vi "Write SA Pin.vi"(8 "error in (no error)":errorcluster, 10 "SA Pin":string, 11 "TDSCDMA_SEM in":refnum<class "TDSCDMA_SEM.lvclass">=refnum) -> (0 "error out":errorcluster, 3 "TDSCDMA_SEM out":refnum<class "TDSCDMA_SEM.lvclass">)   [LabVIEW 2016, in "SeqAuto Evaluations.lvlib" / "TDSCDMA_SEM.lvclass"]
uses:
  TDSCDMA_SEM.lvclass
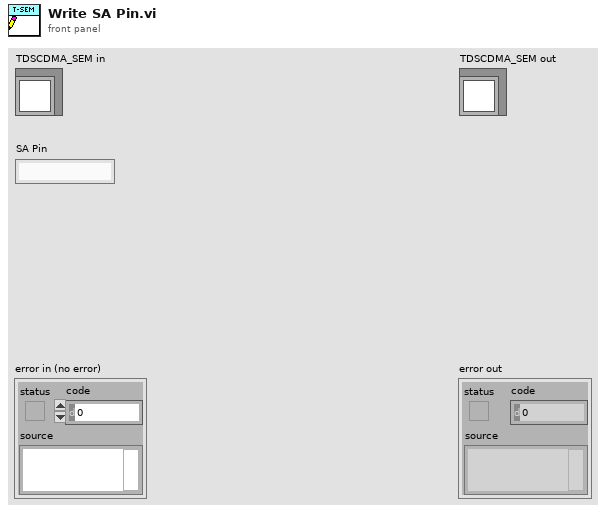
[diagram p1: front panel]
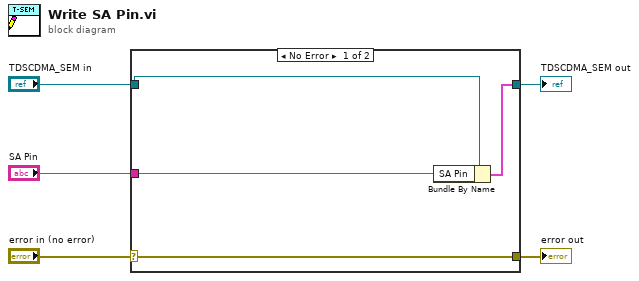
[diagram p0: block diagram]
diagram:
  n1 = case shown="No Error" "error in (no error)" {
    selector: "error in (no error)" -> [w9 w10]
    tunnel: [w9 w10] -> w4
    tunnel: [w7 w11] -> w2
    tunnel: "TDSCDMA_SEM in" -> [w8 w11]
    tunnel: "SA Pin" -> [w6 _]
    frame No Error {
      n2 = Bundle By Name(cluster=w8, "SA Pin"=w6) -> (w7:cluster{})
    }
    frame Error {
    }
  }
  "error out" <- w4
  "TDSCDMA_SEM out" <- w2
